vi "Pair Banner Elements.vi"(10 "boolean switch array in":refnum<vi>[](array[refnum]), 11 "sub vi array in":refnum<vi>[](array[refnum])) -> (3 "banner gui refs":T1[](array[typedef]))   [LabVIEW 2020]
uses:
  GUI References.ctl
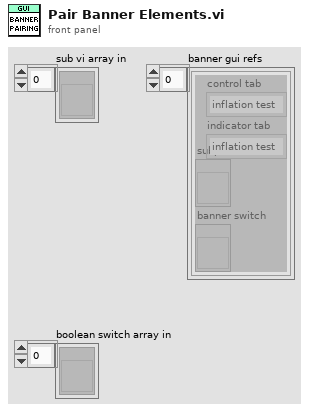
[diagram p1: front panel]
types:
  T1 = typedef "GUI References.ctl" = cluster{"control tab":enum32{"inflation test", "force calibration", "camera calibration", "test equipment"}, "indicator tab":enum32{"inflation test", "force calibration", "camera calibration", "test equipment"}, "subpanel vi":refnum<vi>, "banner switch":refnum<vi>}
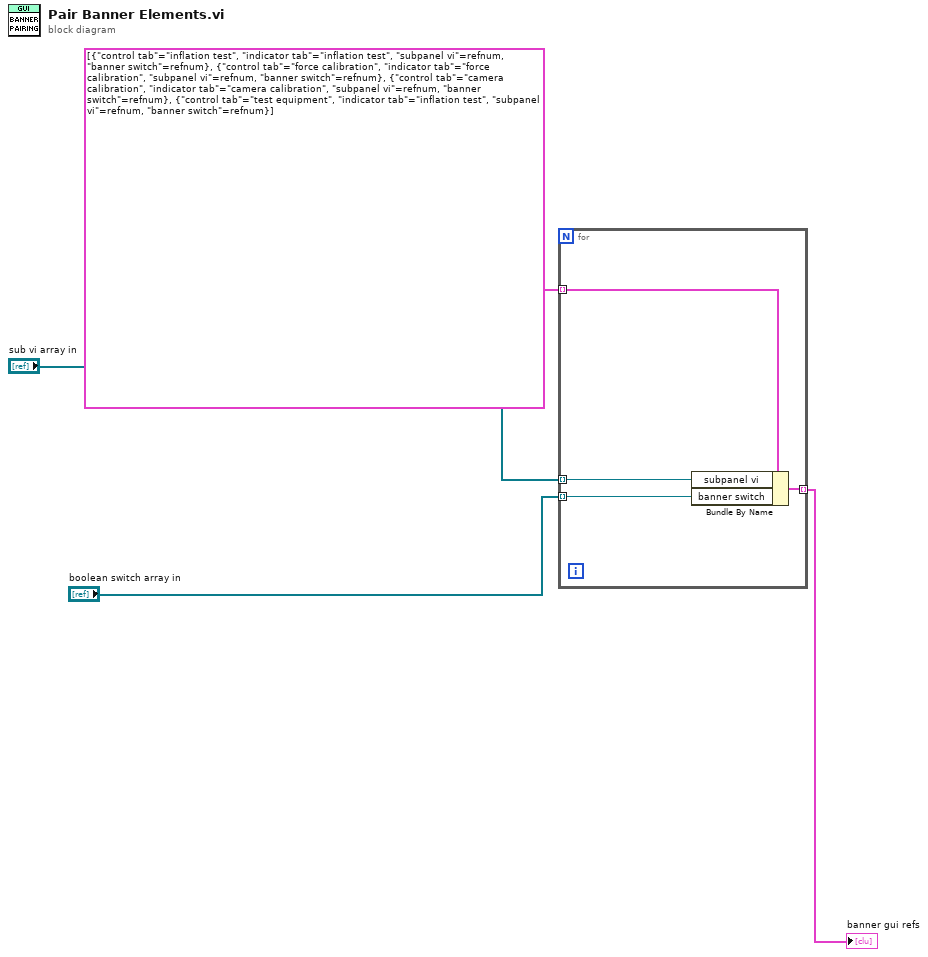
[diagram p0: block diagram]
diagram:
  n1 = for {
    tunnel: T1[] [{"control tab"=enum."inflation test", "indicator tab"=enum."inflation test", "subpanel vi"=refnum, "banner switch"=refnum}, {"control tab"=enum."force calibration", "indicator tab"=enum."force calibration", "subpanel vi"=refnum, "banner switch"=refnum}, {"control tab"=enum."camera calibration", "indicator tab"=enum."camera calibration", "subpanel vi"=refnum, "banner switch"=refnum}, {"control tab"=enum."test equipment", "indicator tab"=enum."inflation test", "subpanel vi"=refnum, "banner switch"=refnum}] -> [w8] mode=indexing
    tunnel: "sub vi array in" -> [w7] mode=indexing
    tunnel: "boolean switch array in" -> [w6] mode=indexing
    tunnel: [w5] -> w4 mode=indexing
    n2 = Bundle By Name(cluster=w8, "subpanel vi"=w7, "banner switch"=w6) -> (w5:T1)
  }
  "banner gui refs" <- w4
